vi "checkLimitSwitchActive.vi"(8 "error in (no error)":errorcluster, 11 "Model in":refnum<class "Model.lvclass">) -> (0 "error out":errorcluster, 3 "Model out":refnum<class "Model.lvclass">)   [LabVIEW 2015]
uses:
  <userlib>/Common/ILC/ILC/ILC.lvclass
  Model.lvclass
panel:
  out "limitSwitchOperatedIsTrue":bool
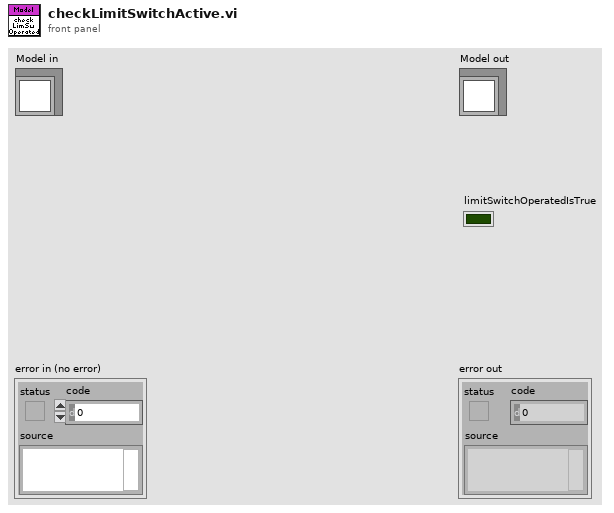
[diagram p1: front panel]
types:
  T1 = typedef "ILCCommon.lvlib/ILCTypedefs.lvlib/InputData.ctl" = cluster{"Input Channels":T2, "Limit Switches":T3, "Tachometer":u16, "SSI Encoder":i32, "ADCs":T4}
  T2 = typedef "ILCCommon.lvlib/ILCConfiguration.lvlib/InputChannels.ctl" = enum16{"Channel 0", "3 Channels", "5 Channels"}
  T3 = typedef "ILCCommon.lvlib/ILCTypedefs.lvlib/LimitSwitches.ctl" = cluster{"1":bool, "2":bool}
  T4 = typedef "ILCCommon.lvlib/ILCTypedefs.lvlib/ADCs.ctl" = cluster{"Ch0":i32, "Ch1":i32, "Ch2":i32, "Ch3":i32, "Ch4":i32}
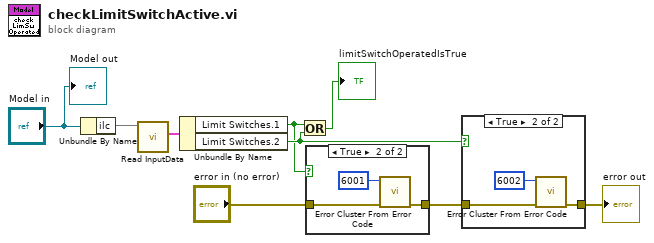
[diagram p0: block diagram]
diagram:
  n1 = Unbundle By Name("Model in") -> ("ilc"=w8)
  n2 = call <userlib>:"Read InputData.vi"("ILC in"=w8) -> ("InputData"=w7:T1)  [unwired: 9 in, 1 out]
  n3 = Unbundle By Name(w7) -> ("Limit Switches.1"=w1:bool, "Limit Switches.2"=w2:bool)
  n4 = Or(x=w1, y=w2) -> (x .or. y?=→"limitSwitchOperatedIsTrue":bool)
  n5 = case shown="True" w1 {
    tunnel: "error in (no error)" -> [w10 w13]
    tunnel: [w10 w12] -> w4
    frame False {
    }
    frame True {
      n6 = call <vilib>:"Error Cluster From Error Code.vi"("error in (no error)"=w13, "error code (0)"=6001) -> ("error out"=w12:errorcluster)  [unwired: 7 in]
    }
  }
  n7 = case shown="True" w2 {
    tunnel: w4 -> [w14 w17]
    tunnel: [w14 w16] -> w3
    frame False {
    }
    frame True {
      n8 = call <vilib>:"Error Cluster From Error Code.vi"("error in (no error)"=w17, "error code (0)"=6002) -> ("error out"=w16:errorcluster)  [unwired: 7 in]
    }
  }
  "error out" <- w3
  "Model out" <- "Model in"
